vi "CalculateContrastofTIFF.vi"(7 "Offset-Konstante":i16=90, 8 "error in":errorcluster, 11 "file path":path) -> (0 "error out":errorcluster, 1 "mean value":dbl, 2 "Waveform Graph":dbl[](graph), 3 "max value":dbl)   [LabVIEW 2011]
uses:
  <vilib>/Analysis/2dsp.llb/Decimate (single shot, DBL).vi
  <vilib>/Analysis/NI_AALPro.lvlib
  <vilib>/Analysis/NI_AALBase.lvlib
panel:
  out "Grid-data (<0: Auto) 2":T1
  in  "Grid-data (<0: Auto)":T1={"Ebenen-Abstand [pix]"=4.13, "Drehwinkel"=19.1}
  out "Numeric":i32
  out "Mean":dbl[](graph)
  in  "x-length":i32=1500
  in  "x-start":i32=500
  in  "y-length":i32=900
  in  "y-start":i32=100
  out "Contrast":dbl[][](graph)
  in  "Boxsize":u16=128
  out "Image":u16[][](graph)
  # "do much lower offset: less correct number but weak signal is dampend"
  # "large>rest"
  # "25,5:4.13\n29: 4.7"
  # "fret6.15/unten -19.1"
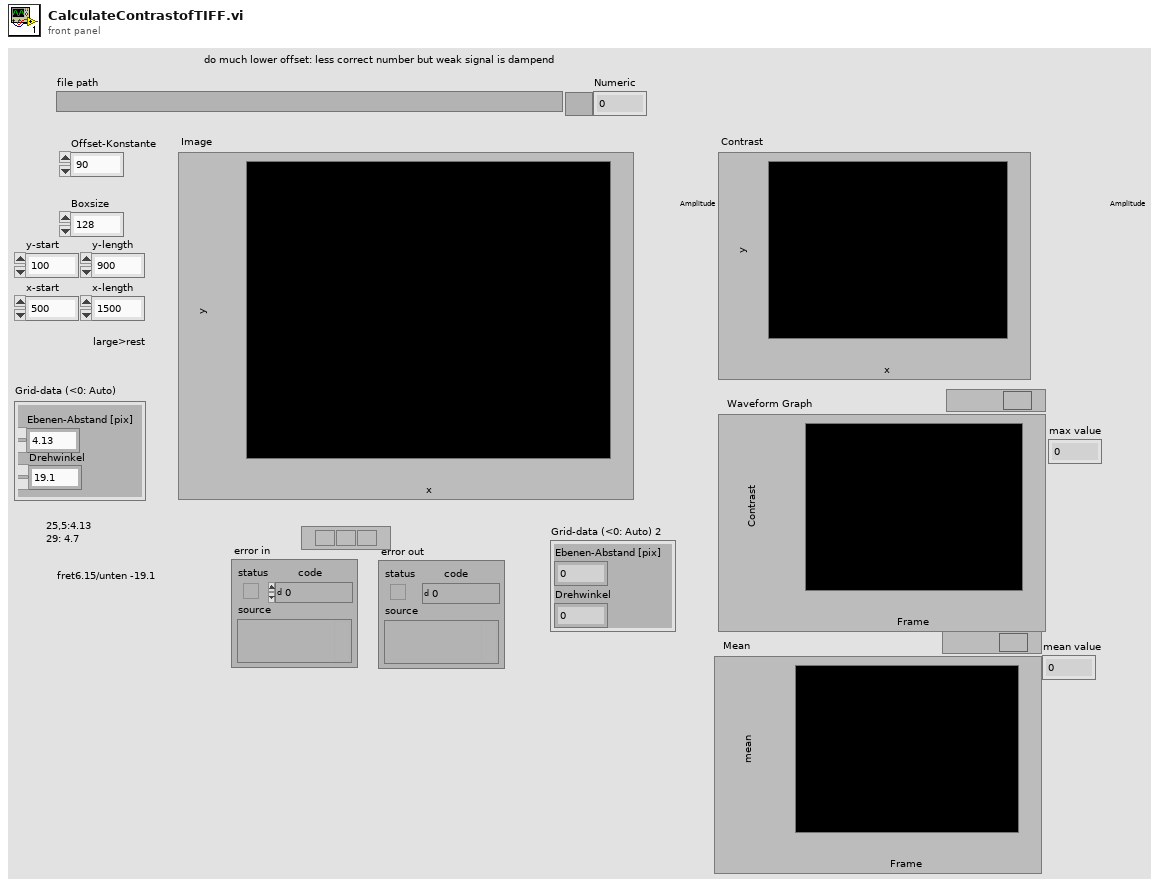
[diagram p1: front panel]
types:
  T1 = cluster{"Ebenen-Abstand [pix]":dbl, "Drehwinkel":dbl}
  T2 = cluster{"Tiff refnum":refnum<file>, "BigTiff,Endian":u16}
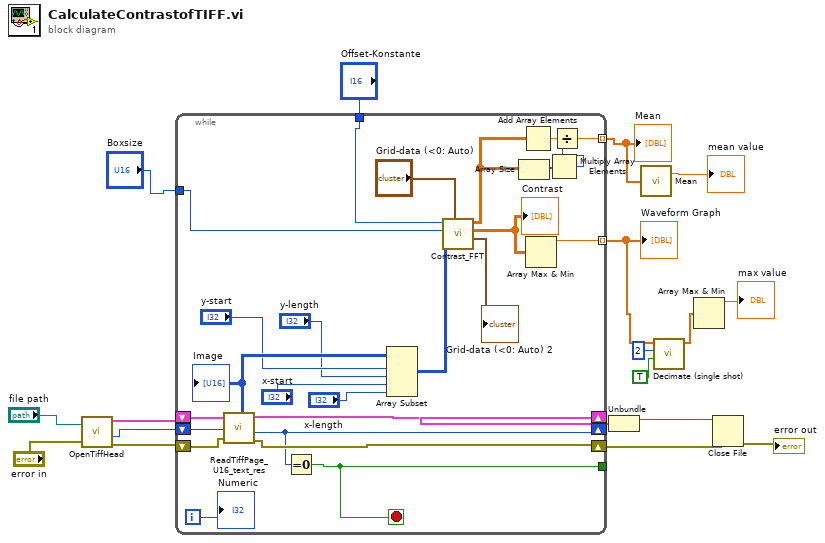
[diagram p0: block diagram]
diagram:
  n1 = call "OpenTiffHead.vi"("file path"="file path", "error in"="error in") -> ("TIFF file"=w15:T2, "first Diroffset"=w16:u64, "error out"=w14:errorcluster)  [unwired: 1 in]
  n2 = while {
    shift-right: [w34] -> _
    shift-left: w16 -> [w43]
    shift-right: [w39] -> w11
    shift-left: w15 -> [w42]
    shift-right: [w40] -> w10
    shift-left: w14 -> [w41]
    tunnel: [w38] -> _
    tunnel: "Boxsize" -> [w26]
    tunnel: "Offset-Konstante" -> [w37]
    tunnel: [w35] -> w6 mode=indexing
    tunnel: [w27] -> w2 mode=indexing
    i -> [w25]
    stop <- w38 stop-if-true
    n3 = call "ReadTiffPage_U16_text_res.vi"("TIFF file"=w42, "IFDoffset"=w43, "error in"=w41) -> ("TIFF file out"=w39:T2, "16-bit pixmap"=w23:u16[][], "Next offset"=w34:i64, "error out"=w40:errorcluster)  [unwired: 2 in, 2 out]
    "Image" <- w23
    n4 = Equal To 0?(x=w34) -> (x = 0?=w38:bool)
    n5 = Array Subset(array=w23, index (row)="y-start", length (row)="y-length", index (col)="x-start", length (col)="x-length") -> (w32:u16[][])
    n6 = call "Contrast_FFT.vi"("Grid-data (<0: Auto)"="Grid-data (<0: Auto)", "Image in"=w32, "Boxsize"=w26, "Offset-Konstante"=w37) -> ("Grid-data (<0: Auto) 2"=→"Grid-data (<0: Auto) 2":T1, "Contrast out"=w36:dbl[][], "Mean out"=w31:dbl[][])  [unwired: 5 in]
    "Contrast" <- w36
    n7 = Array Size(array=w31) -> (size(s)=w30:i32[])
    n8 = Add Array Elements(numeric array=w31) -> (sum=w29:dbl)
    n9 = Array Max & Min(array=w36) -> (max value=w35:dbl)  [unwired: 3 out]
    n10 = Multiply Array Elements(1:w30) -> (0:w28:i32)
    n11 = Divide(x=w29, y=w28) -> (x/y=w27:dbl)
    "Numeric" <- w25
  }
  "Waveform Graph" <- w6
  "Mean" <- w2
  n12 = Unbundle(w11) -> ("Tiff refnum"=w13:refnum<file>)  [unwired: 1 out]
  n13 = call <vilib>:"Mean.vi"("X"=w2) -> ("mean"=→"mean value":dbl)  [unwired: 1 out]
  n14 = call-poly <vilib>:"Decimate (single shot).vi"("averaging"=TRUE, "decimating factor"=2, "X"=w6) -> ("Decimated Array"=w3:dbl[])  [unwired: 7 in, 1 out]
  n15 = Array Max & Min(array=w3) -> (max value=→"max value":dbl)  [unwired: 3 out]
  n16 = Close File(refnum=w13, error in=w10) -> (error out=→"error out":errorcluster)  [unwired: 1 out]
